vi "Coll_Det_Example.vi"() -> ()   [LabVIEW 2011]
uses:
  SObject.ctl
  Vector3D.ctl
panel:
  out "error out":errorcluster
  in  "stop":bool
  out "Collision Detected Array":bool[](array[boolean])
  in  "Moving Positions":T1
  in  "Data Folder":path=path "C:/EnFlo_Data_Local/2012/Aero_Tunnel/Nick_Martin/Preferences/Traverse_Space_ColDet"
  in  "Lock to 60Hz?":bool
  in  "Height":i32=600
  in  "Width":i32=800
  in  "Graphics Driver Type":T2(ring)=enum."DirectX 9"
  in  "Camera Type":T3(ring)=enum."Standard Camera"
  out "FPS":i32=629
  out "SepDistance":T4[](array[typedef])=[{"X"=-12.215232849121094, "Y"=5.8577728271484375, "Z"=21.565397262573242}, {"X"=0.2394256591796875, "Y"=-15.688332557678223, "Z"=-24.610620498657227}, {"X"=126.86971282958984, "Y"=10.406116485595703, "Z"=28.3343563079834}, {"X"=-6.2993011474609375, "Y"=34.38507080078125, "Z"=60.643470764160156}]
  in  "Alpha":dbl=0.5
  in  "Probe Position":T1
  in  "Color":u32(colorbox)=12763842
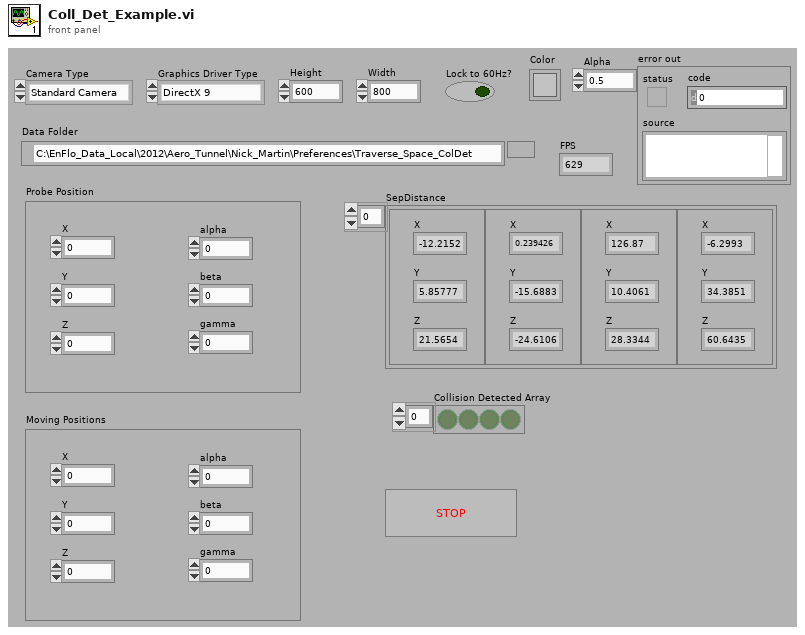
[diagram p1: front panel]
types:
  T1 = typedef "SObject.ctl" = cluster{"X":dbl, "Y":dbl, "Z":dbl, "alpha":dbl, "beta":dbl, "gamma":dbl}
  T2 = enum32{"No Driver (NULL)", "Software Driver", "Burnings Video", "DirectX 8", "DirectX 9", "OpenGL", "Count"}
  T3 = enum32{"Fixed Camera", "Standard Camera", "Flying Camera"}
  T4 = typedef "Vector3D.ctl" = cluster{"X":dbl, "Y":dbl, "Z":dbl}
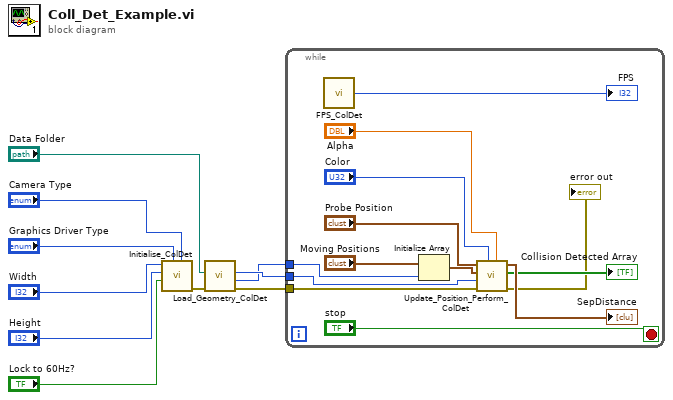
[diagram p0: block diagram]
diagram:
  n1 = call "Initialise_ColDet.vi"("Camera Type"="Camera Type", "Graphics Driver Type"="Graphics Driver Type", "Lock to 60Hz?"="Lock to 60Hz?", "Height"="Height", "Width"="Width") -> ("error out"=w10:errorcluster)  [unwired: 6 in]
  n2 = call "Load_Geometry_ColDet.vi"("error in"=w10, "Data Folder"="Data Folder") -> ("error out"=w9:errorcluster, "Number Moving"=w1:i32, "Number Static"=w2:i32)  [unwired: 7 in]
  n3 = while {
    tunnel: w9 -> [w23]
    tunnel: w1 -> [w17]
    tunnel: w2 -> [w22]
    stop <- "stop" stop-if-true
    n4 = call "FPS_ColDet.vi"() -> ("Current FPS"=→"FPS":i32)  [unwired: 6 in]
    n5 = Initialize Array("Moving Positions", w17) -> (w16:T1[])
    n6 = call "Update_Position_Perform_ColDet.vi"("Background Alpha"="Alpha", "Background Color"="Color", "error in"=w23, "Number Static"=w22, "Moving Position Array"=w16, "Probe Position"="Probe Position") -> ("error out"=→"error out":errorcluster, "Collision Detected Array"=→"Collision Detected Array":bool[], "Separation Distance Array"=→"SepDistance":T4[])  [unwired: 3 in]
  }
